vi "MVA Test.vi"() -> ()   [LabVIEW 2012]
uses:
  <vilib>/Utility/miscctls.llb/LVDateTimeRec.ctl
  <vilib>/addons/database/Connection.llb/DB Tools Open Connec (String).vi
  <vilib>/addons/database/Connection.llb/Conn Execute.vi
  <vilib>/addons/database/Recordset.llb/Rec Fetch Recordset Data (R).vi
  <vilib>/addons/database/Recordset.llb/Rec Destroy - Connection.vi
  <vilib>/Analysis/baseanly.llb/Mean (DBL).vi
  <vilib>/LVH/i3 JSON/JSON Parsing/Get Array Value at Index Files/Get Array Value at Index - Object.vi
  <vilib>/LVH/i3 JSON/JSON Parsing/Get Object Parameter Files/Get Object Parameter - Numeric.vi
  <vilib>/LVH/i3 JSON/JSON Parsing/Get Object Parameter Files/Get Object Parameter - String.vi
  <vilib>/addons/database/_DB Variant To Data/Database Variant To Data.xnode
  <vilib>/httpClient/LabVIEWHTTPClient.lvlib
  <vilib>/LVH/i3 JSON/i3-json.lvlib
  <vilib>/addons/database/NI_Database_API.lvlib
  <vilib>/Analysis/NI_AALBase.lvlib
panel:
  out "mean number of MVA CTS":dbl format="%0.2f"
  out "Main Plot":cluster{dbl[], dbl[]}[](graph)
  in  "End Time Stamp":timestamp=timestamp(3468686517.2101927 s since 1904-01-01) format="%<%m/%d/%Y>T"
  in  "Start Time Stamp":timestamp=timestamp(3439915312.43992 s since 1904-01-01) format="%<%m/%d/%Y>T"
  in  "password":string="password123%%%"
  in  "userID":string="john"
  out "headers":string
  in  "Monroe url":string="http://mcsafetyfeed.org/api/counts.php?type=mva"
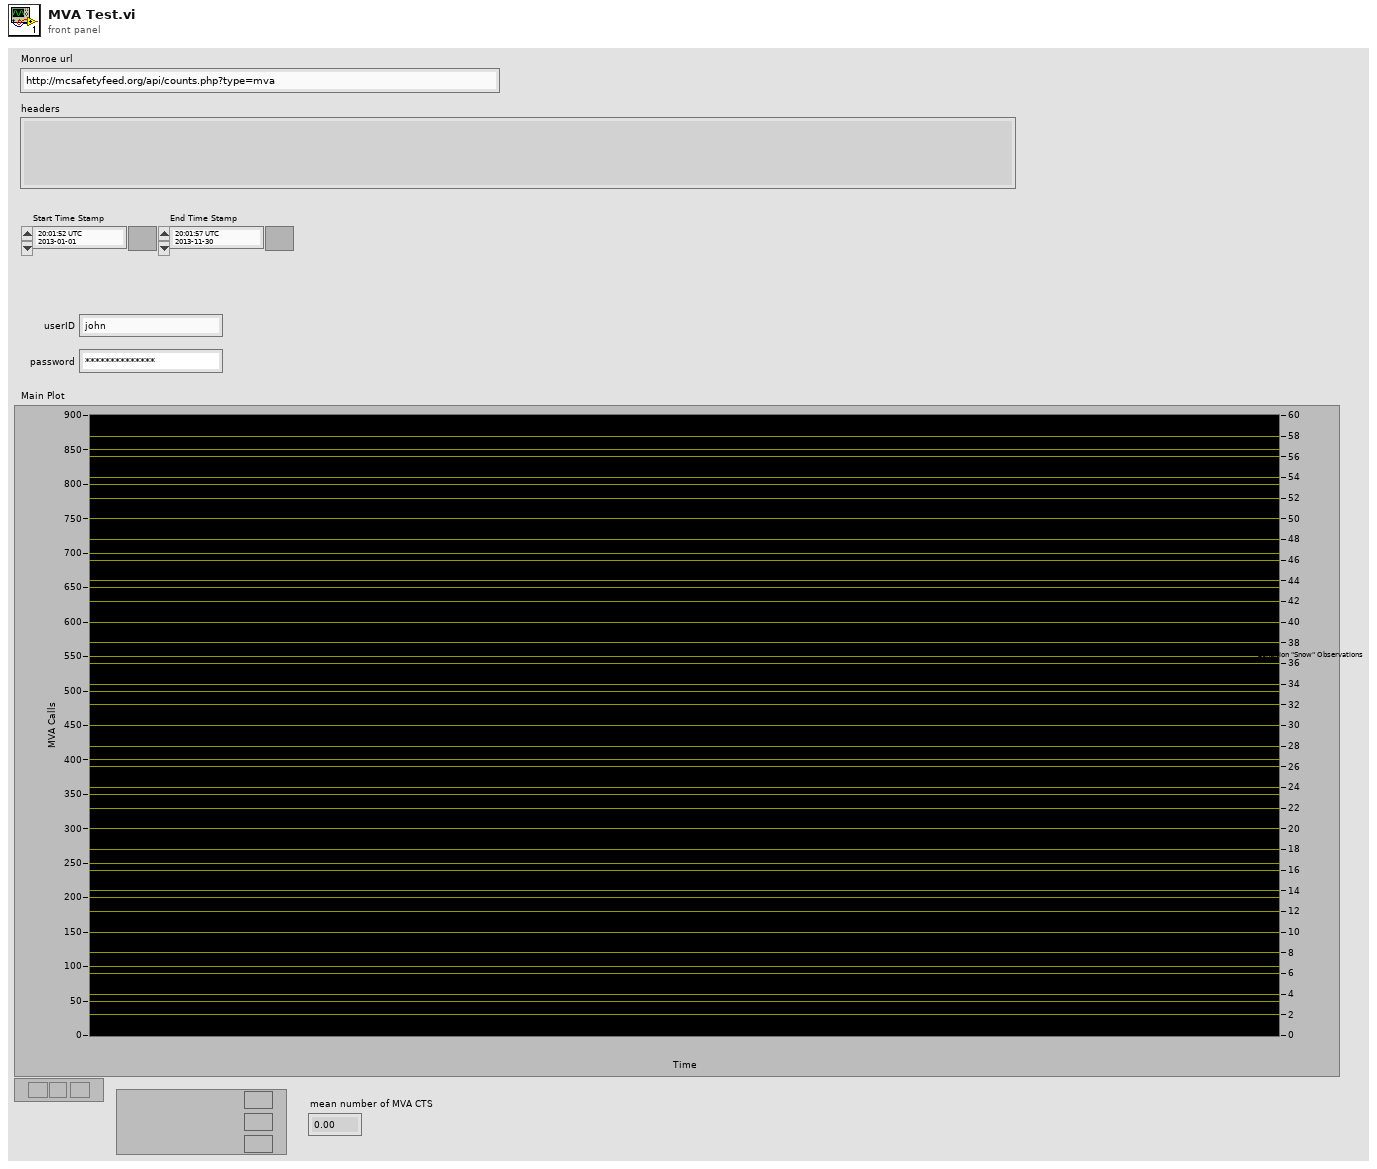
[diagram p1: front panel]
types:
  T1 = typedef "LabVIEWHTTPClient.lvlib/ClientHandle.ctl" = refnum<k1>
  T2 = typedef "LVDateTimeRec.ctl" = cluster{"fractional second":dbl, "second":i32, "minute":i32, "hour":i32, "day of month":i32, "month":i32, "year":i32, "day of week":i32, "day of year":i32, "DST":i32}
  T3 = typedef "NI_Database_API.lvlib/Conn ObjectReference.ctl" = refnum<k1>
  T4 = typedef "NI_Database_API.lvlib/Rec ObjectReference.ctl" = refnum<k1>
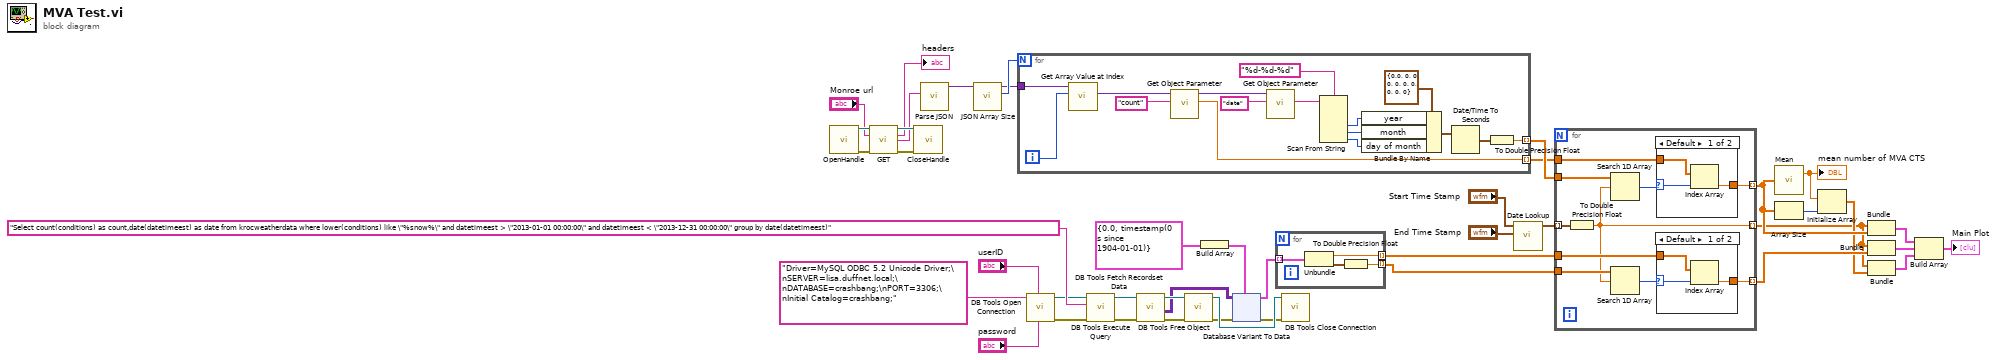
[diagram p0: block diagram]
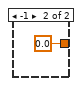
[diagram p2: hidden frame]
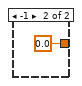
[diagram p3: hidden frame]
diagram:
  n1 = call <vilib>:"OpenHandle.vi"() -> ("client handle out"=w10:T1, "error out"=w9:errorcluster)  [unwired: 14 in]
  n2 = call <vilib>:"GET.vi"("client handle"=w10, "url"="Monroe url", "error in (no error)"=w9) -> ("client handle out"=w7:T1, "headers"=→"headers":string, "body"=w4:string, "error out"=w8:errorcluster)  [unwired: 9 in]
  n3 = call <vilib>:"CloseHandle.vi"("client handle"=w7, "error in (no error)"=w8) -> ()  [unwired: 13 in, 1 out]
  n4 = call <vilib>:"Parse JSON.vi"("JSON String"=w4) -> ("JSON Tree"=w3:variant)  [unwired: 7 in, 3 out]
  n5 = call <vilib>:"JSON Array Size.vi"("JSON Tree In (JSON Array)"=w3) -> ("Array Size"=w2:i32, "JSON Tree Passthrough (JSON Array)"=w1:variant)  [unwired: 8 in, 1 out]
  n6 = for {
    N: w2 -> [_]
    tunnel: w1 -> [w60]
    tunnel: [w46] -> w23 mode=indexing
    tunnel: [w45] -> w22 mode=indexing
    i -> [w59]
    n7 = call-poly <vilib>:"Get Array Value at Index.vi"("Index"=w59, "JSON Tree In (JSON Array)"=w60) -> ("JSON Object"=w58:variant)  [unwired: 6 in, 3 out]
    n8 = call-poly <vilib>:"Get Object Parameter.vi"("Parameter Name"="count", "JSON Tree In (JSON Object)"=w58) -> ("Double Value"=w45:dbl, "JSON Tree Out Passthrough"=w56:variant)  [unwired: 6 in, 2 out]
    n9 = call-poly <vilib>:"Get Object Parameter.vi"("Parameter Name"="date", "JSON Tree In (JSON Object)"=w56) -> ("String Value"=w54:string)  [unwired: 6 in, 3 out]
    n10 = Scan From String(format string="%d-%d-%d", input string=w54) -> (output 1=w51:i32, output 2=w50:i32, output 3=w49:i32)  [unwired: 5 in, 3 out]
    n11 = Bundle By Name(cluster=T2 {"fractional second"=0.0, "second"=0, "minute"=0, "hour"=0, "day of month"=0, "month"=0, "year"=0, "day of week"=0, "day of year"=0, "DST"=0} ("date time rec"), "year"=w51, "month"=w50, "day of month"=w49) -> (w48:T2)
    n12 = Date/Time To Seconds(2:w48) -> (0:w47:timestamp)  [unwired: 1 in]
    n13 = To Double Precision Float(number=w47) -> (double precision float=w46:dbl)
  }
  n14 = call-poly <vilib>:"DB Tools Open Connection.vi"("password"="password", "userID"="userID", "connection information"="Driver=MySQL ODBC 5.2 Unicode Driver;\nSERVER=lisa.duffnet.local;\nDATABASE=crashbang;\nPORT=3306;\nInitial Catalog=crashbang;") -> ("error out"=w32:errorcluster, "connection reference"=w33:T3)  [unwired: 5 in]
  n15 = call-poly <vilib>:"DB Tools Execute Query.vi"("error in (no error)"=w32, "SQL query"="Select count(conditions) as count,date(datetimeest) as date from krocweatherdata where lower(conditions) like \"%snow%\" and datetimeest > \"2013-01-01 00:00:00\" and datetimeest < \"2013-12-31 00:00:00\" group by date(datetimeest)", "connection reference"=w33) -> ("error out"=w42:errorcluster, "recordset reference"=w41:T4)  [unwired: 5 in]
  n16 = call-poly <vilib>:"DB Tools Fetch Recordset Data.vi"("error in (no error)"=w42, "recordset reference"=w41) -> ("error out"=w36:errorcluster, "recordset data"=w37:variant[][], "recordset reference out"=w40:T4)  [unwired: 3 in]
  n17 = call-poly <vilib>:"DB Tools Free Object.vi"("error in (no error)"=w36, "recordset reference"=w40) -> ("error out"=w35:errorcluster, "connection reference"=w39:T3)  [unwired: 8 in]
  n18 = Build Array(cluster{dbl, timestamp} {0.0, timestamp(0 s since 1904-01-01)}) -> (w30:cluster{dbl, timestamp}[])
  n19 = xnode "Database Variant To Data"("database variant"=w37, "error in (no error)"=w35, "type"=w30) -> ("data"=w29:cluster{dbl, timestamp}[], "error out"=w34:errorcluster)
  n20 = for {
    tunnel: w29 -> [w64] mode=indexing
    tunnel: [w62] -> w25 mode=indexing
    tunnel: [w61] -> w24 mode=indexing
    n21 = Unbundle(w64) -> (w61:dbl, w63:timestamp)
    n22 = To Double Precision Float(number=w63) -> (double precision float=w62:dbl)
  }
  n23 = call <vilib>:"DB Tools Close Connection.vi"("error in (no error)"=w34, "connection reference"=w39) -> ()  [unwired: 5 in, 1 out]
  n24 = call "Date Lookup.vi"("End Time Stamp"="End Time Stamp", "Start Time Stamp"="Start Time Stamp") -> ("DateTime Array"=w26:timestamp[])  [unwired: 8 in, 1 out]
  n25 = for {
    tunnel: w26 -> [w74] mode=indexing
    tunnel: w25 -> [w69]
    tunnel: w24 -> [w70]
    tunnel: w23 -> [w73]
    tunnel: w22 -> [w71]
    tunnel: [w67] -> w16 mode=indexing
    tunnel: [w66] -> w21 mode=indexing
    tunnel: [w65] -> w13 mode=indexing
    n26 = To Double Precision Float(number=w74) -> (double precision float=w65:dbl)
    n27 = Search 1D Array(1D array=w73, element=w65) -> (index of element=w72:i32)  [unwired: 1 in]
    n28 = Search 1D Array(1D array=w69, element=w65) -> (index of element=w68:i32)  [unwired: 1 in]
    n29 = case shown="Default" w72 {
      selector: w72 -> [w80 _]
      tunnel: w71 -> [w81 _]
      tunnel: [w79 0.0 ("Double Value")] -> w67
      frame Default {
        n30 = Index Array(array=w81, index=w80) -> (element=w79:dbl)
      }
      frame -1 {
      }
    }
    n31 = case shown="Default" w68 {
      selector: w68 -> [w76 _]
      tunnel: w70 -> [w77 _]
      tunnel: [w75 0.0 ("Double Value")] -> w66
      frame Default {
        n32 = Index Array(array=w77, index=w76) -> (element=w75:dbl)
      }
      frame -1 {
      }
    }
  }
  n33 = call-poly <vilib>:"Mean.vi"("X"=w16) -> ("mean"=w17:dbl)  [unwired: 1 out]
  "mean number of MVA CTS" <- w17
  n34 = Array Size(array=w16) -> (size(s)=w15:i32)
  n35 = Initialize Array(w17, w15) -> (w14:dbl[])
  n36 = Bundle(w13, w16) -> (w20:cluster{dbl[], dbl[]})  [unwired: 1 in]
  n37 = Bundle(w13, w21) -> (w19:cluster{dbl[], dbl[]})  [unwired: 1 in]
  n38 = Bundle(w13, w14) -> (w12:cluster{dbl[], dbl[]})  [unwired: 1 in]
  n39 = Build Array(w20, w19, w12) -> (→"Main Plot":cluster{dbl[], dbl[]}[])
